vi "Template No Block Diagram VI.vi"(8 "error in (no error)":errorcluster) -> (0 "error out":errorcluster)   [LabVIEW 2013]
doc: "Statnett PMU Reference Library Template VI with no Block Diagram"
panel:
  # "INPUT"
  # "INTERMEDIATE"
  # "OUTPUT"
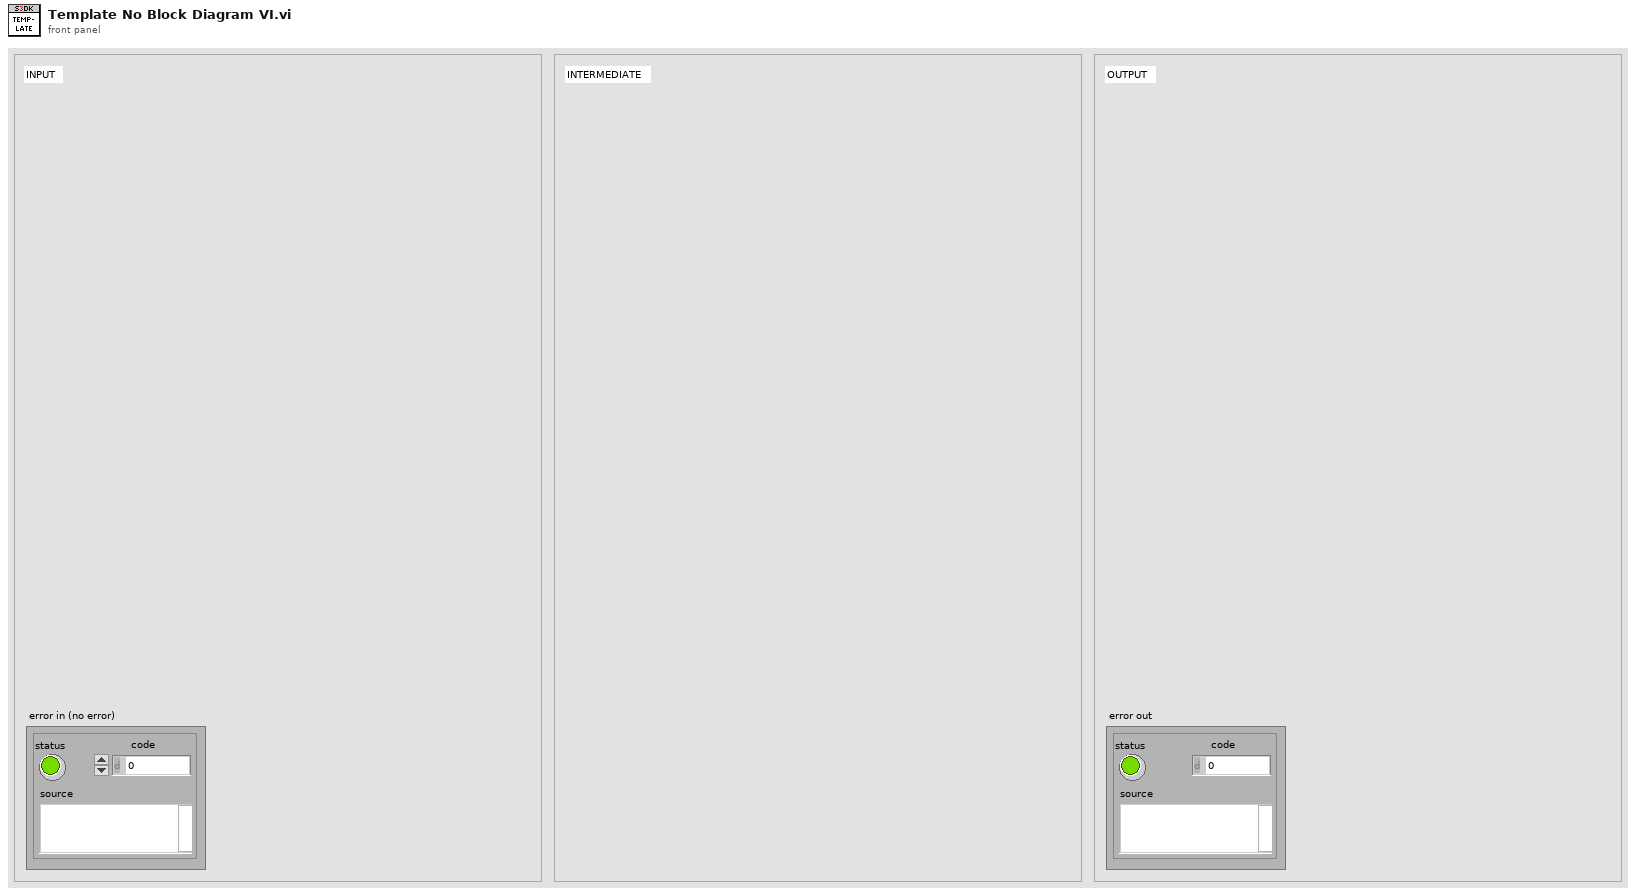
[diagram p1: front panel]
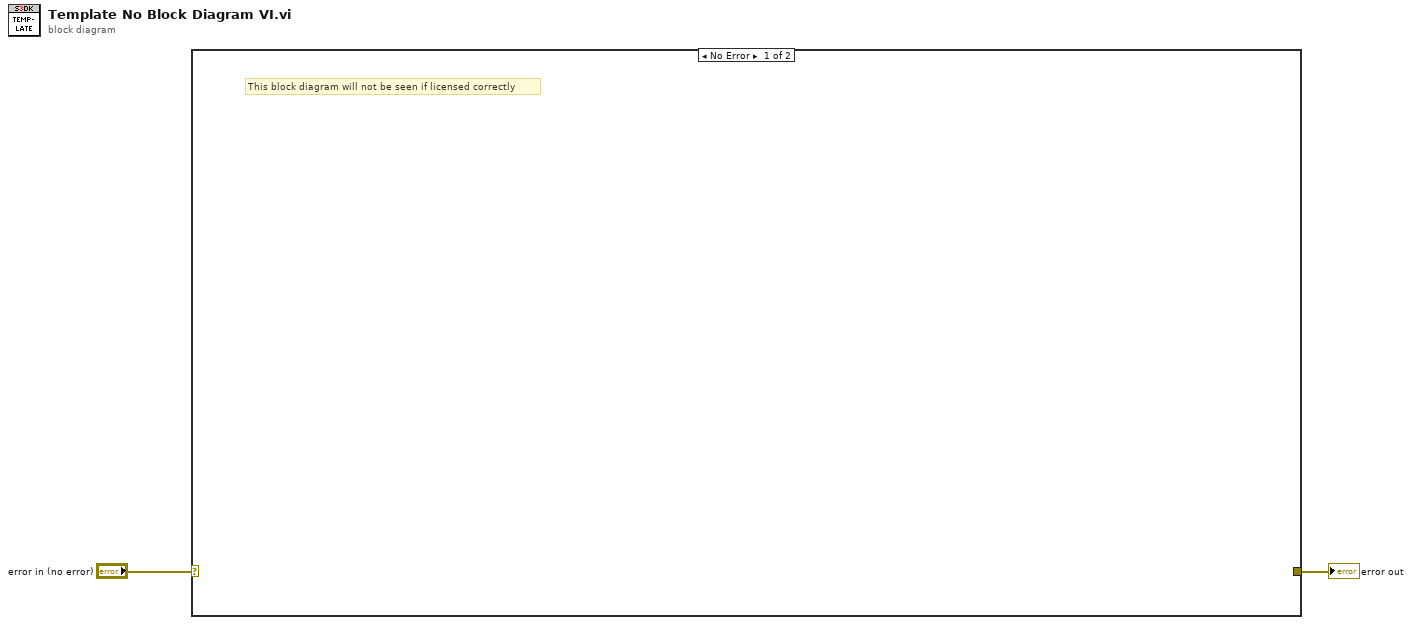
[diagram p0: block diagram]
diagram:
  n1 = case shown="No Error" "error in (no error)" {
    selector: "error in (no error)" -> [_ w3]
    tunnel: [_ w3] -> w1
    frame No Error {
      # "This block diagram will not be seen if licensed correctly"
    }
    frame Error {
    }
  }
  "error out" <- w1
